vi "SA_Selected_Solution.vi"(7 "Perturbation Method":T1=enum."NonRedundantSwap", 8 "error in (no error)":errorcluster, 9 "Schedule In":u16[](array[numeric]), 10 "GA.lvclass":refnum<class "GA.lvclass">, 11 "OSSP_Problem in":refnum<class "OSSP_Problem.lvclass">) -> (0 "error out":errorcluster, 1 "Schedule Out":u16[](array[numeric]), 2 "OSSP_Problem out":refnum<class "OSSP_Problem.lvclass">, 3 "GA out":refnum<class "GA.lvclass">, 4 "Fitness":i16)   [LabVIEW 2013]
uses:
  Classes/GA.lvclass
  Classes/OSSP_Problem.lvclass
  Classes/SA_Class/Controls/Perturbation Method.ctl
  Classes/SA.lvclass
  SA/Controls/States_SA.ctl
  Classes/OSSP_Problem.lvclass/OSSP_Problem.ctl
  Classes/GA.lvclass/GA.ctl
  Classes/SA_Class/Controls/CoolingScheme.ctl
  Classes/SA.lvclass/SA.ctl
  Classes/SA_Class/Controls/Solution_SA.ctl
  Classes/GanntChart_Class/Operation to Machine Job Tuple.vi
  Classes/GanntChart_Class/Check Other Machines for Schedule Time.vi
  Classes/GanntChart_Class/Schedule Job.vi
  Classes/GanntChart_Class/Find Gaps on Particular Machine.vi
  Classes/GanntChart_Class/Increment Number of Jobs on Machine.vi
  Classes/GanntChart_Class/Find Job On Other Machines.vi
  Classes/GanntChart.lvclass
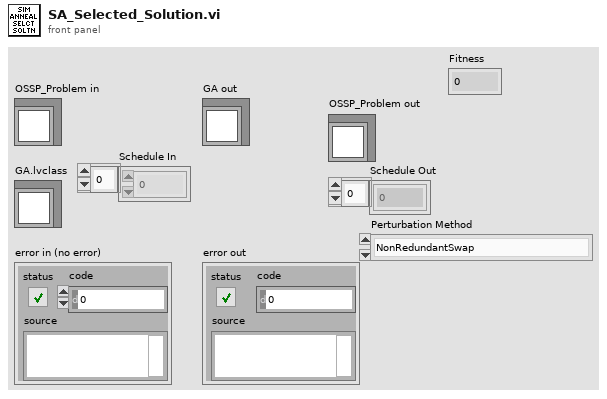
[diagram p1: front panel]
types:
  T1 = typedef "SA.lvclass/Perturbation Method.ctl" = enum16{"Simple Swap", "Insert", "NonRedundantSwap", "Job Order Swap", "Machine Order Swap", "Machine&Job Order Swap", "Critical Path Swap"}
  T2 = typedef "States_SA.ctl" = enum16{"Init", "Read Problem", "Sort Problem", "Generate and Evaluate Current Solution", "Perturb Cur Solution and Eval New Solution", "Make Decision", "Keep Track of Best Solution", "Cool", "Output Final Solution", "Stop"}
  T3 = typedef "Scheduler Type.ctl" = enum16{"Non Delay Scheduler", "GT Active Scheduler", "FIFO Scheduler"}
  T4 = typedef "Objective.ctl" = enum16{"Makespan", "Total Tardiness"}
  T5 = typedef "SA.lvclass/CoolingScheme.ctl" = enum16{"Linear", "Geometric"}
  T6 = typedef "SA.lvclass/Solution_SA.ctl" = cluster{"Schedule":u16[], "Fitness":i16}
  T7 = typedef "GanntChart_Element.ctl" = cluster{"Operation Number":i32, "Job Number":i32, "Start Time":i32, "Procesing Time":u16, "End Time":i32}
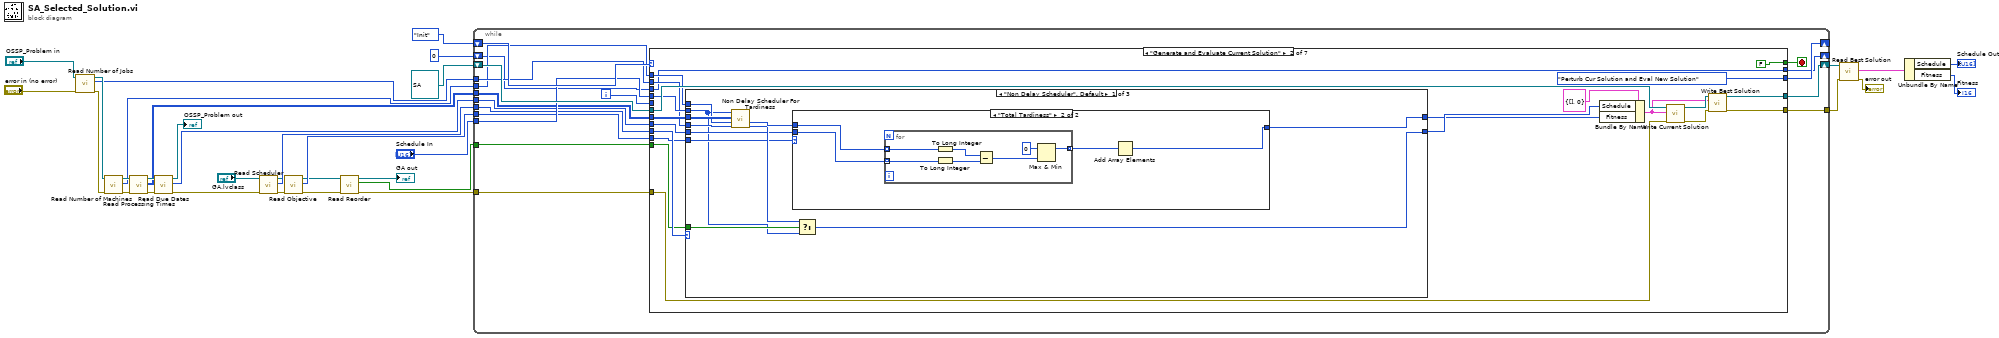
[diagram p0: block diagram]
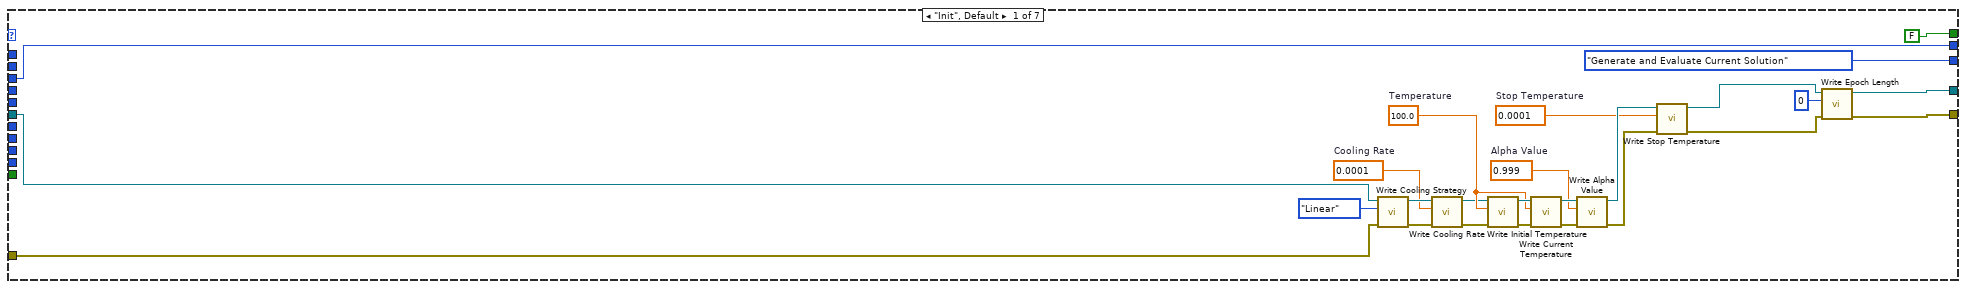
[diagram p2: hidden frame]
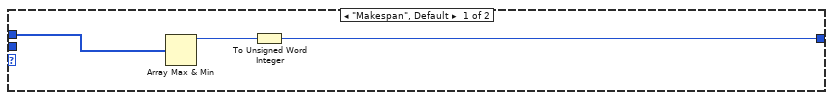
[diagram p3: hidden frame]
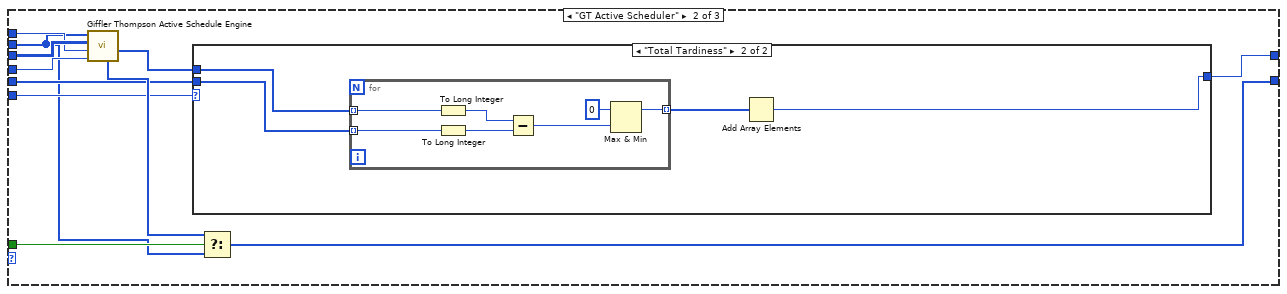
[diagram p4: hidden frame]
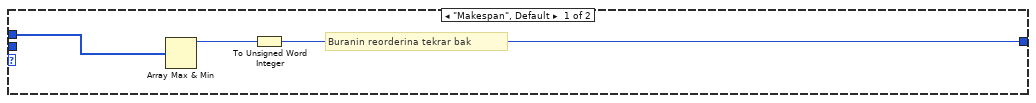
[diagram p5: hidden frame]
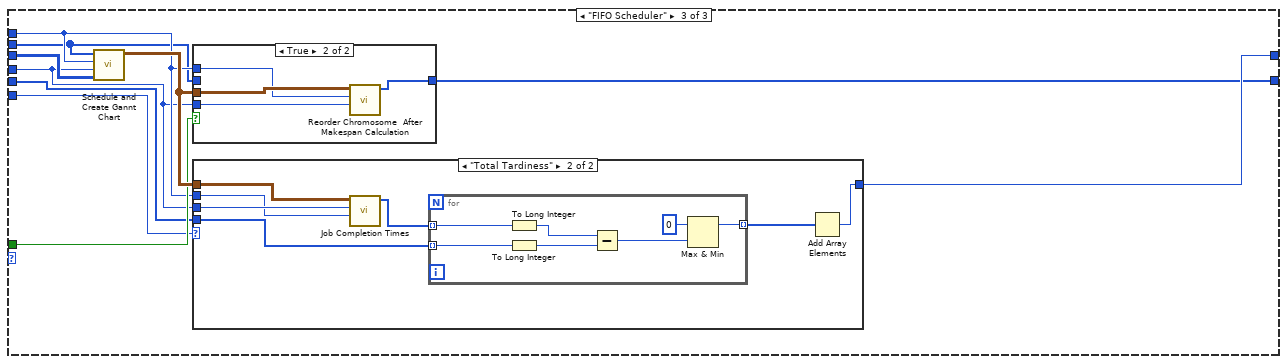
[diagram p6: hidden frame]
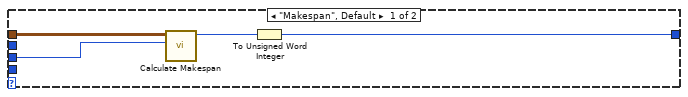
[diagram p8: hidden frame]
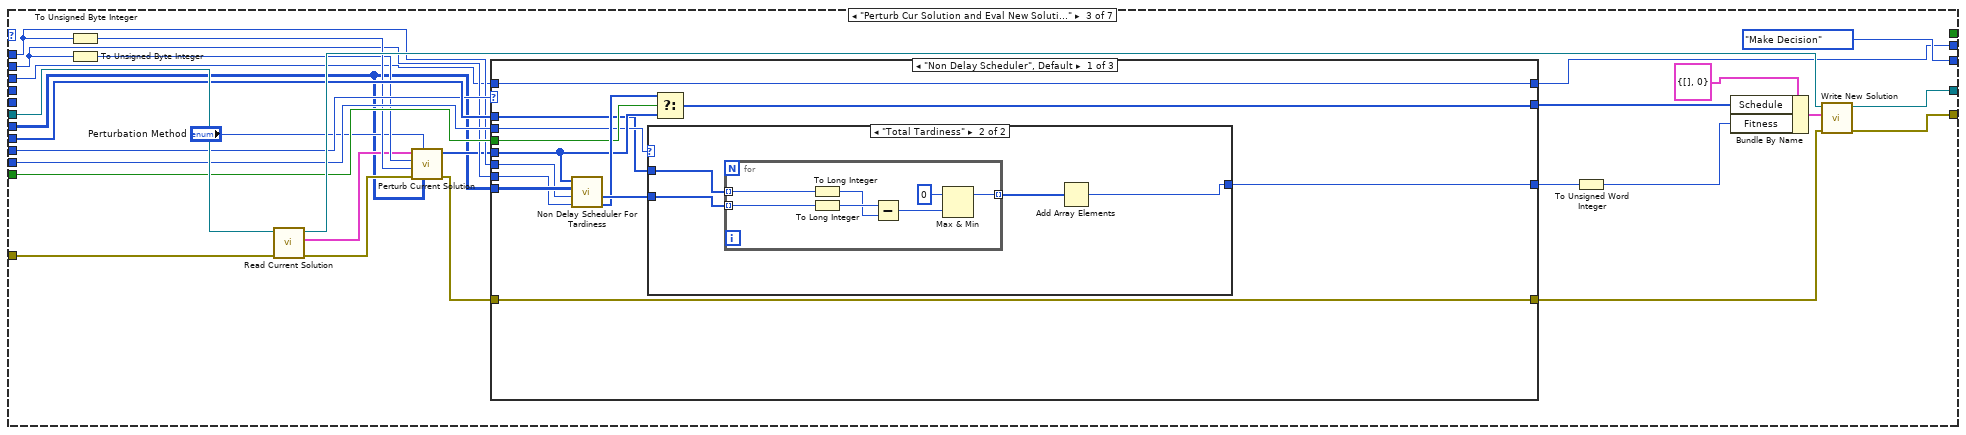
[diagram p9: hidden frame]
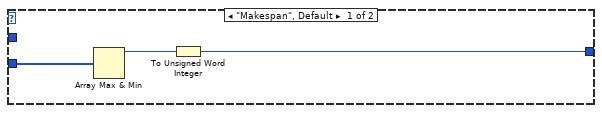
[diagram p10: hidden frame]
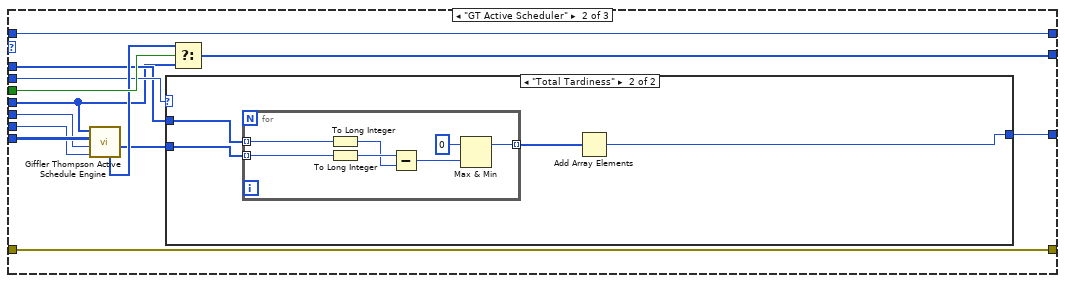
[diagram p11: hidden frame]
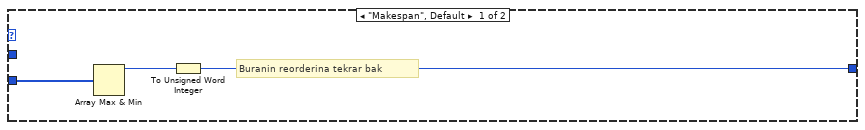
[diagram p12: hidden frame]
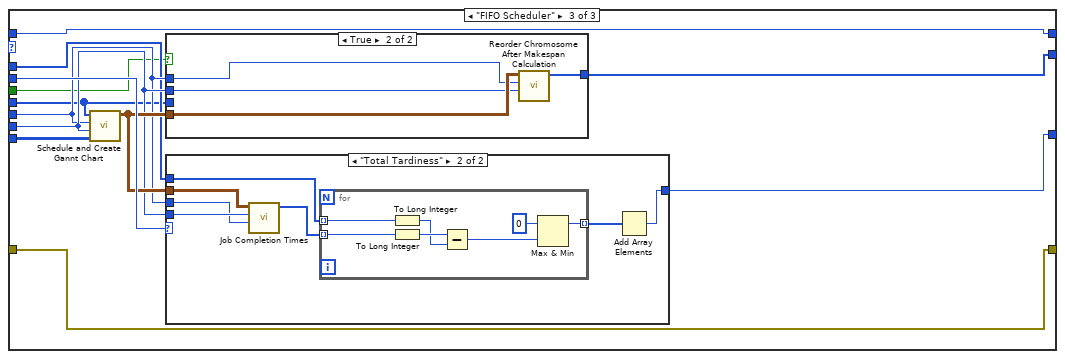
[diagram p13: hidden frame]
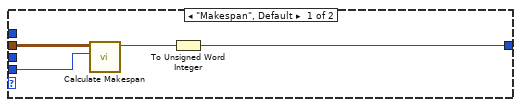
[diagram p15: hidden frame]
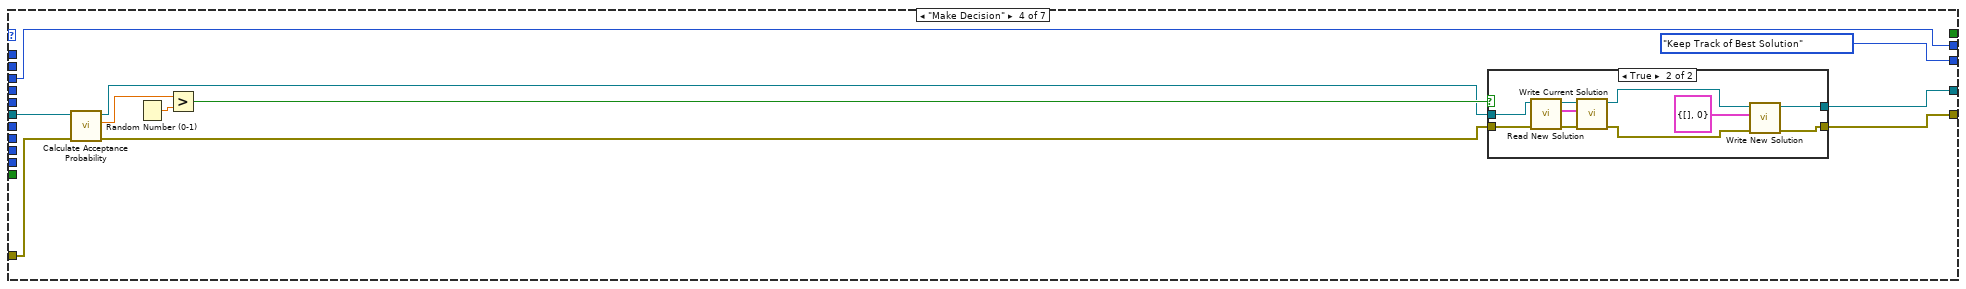
[diagram p16: hidden frame]
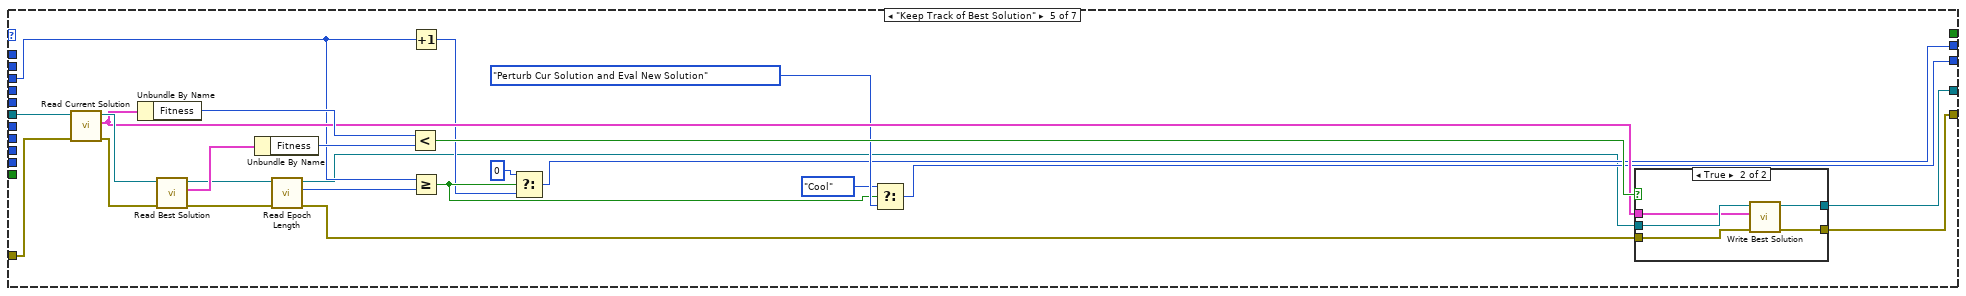
[diagram p18: hidden frame]
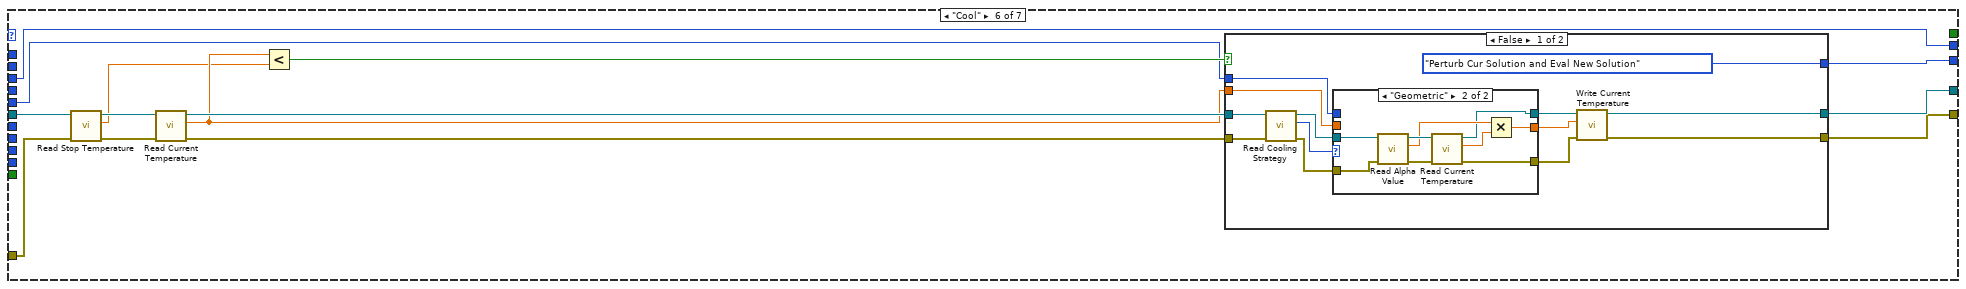
[diagram p20: hidden frame]
diagram:
  n1 = call-dynamic "Read Number of Jobs.vi"("error in (no error)"="error in (no error)", "OSSP_Problem in"="OSSP_Problem in") -> ("error out"=w25:errorcluster, "Number of Jobs"=w29:i32, "OSSP_Problem out"=w31:refnum<class "OSSP_Problem.lvclass">)  [unwired: 7 in]
  n2 = call-dynamic "Read Number of Machines.vi"("error in (no error)"=w25, "OSSP_Problem in"=w31) -> ("error out"=w24:errorcluster, "Number of Machines"=w28:i32, "OSSP_Problem out"=w30:refnum<class "OSSP_Problem.lvclass">)  [unwired: 7 in]
  n3 = call-dynamic "Read Processing Times.vi"("error in (no error)"=w24, "OSSP_Problem in"=w30) -> ("error out"=w23:errorcluster, "Processing Times"=w9:u16[][], "OSSP_Problem out"=w22:refnum<class "OSSP_Problem.lvclass">)  [unwired: 7 in]
  n4 = call "Read Due Dates.vi"("error in (no error)"=w23, "OSSP_Problem in"=w22) -> ("error out"=w20:errorcluster, "Due Dates"=w21:u16[], "OSSP_Problem out"=→"OSSP_Problem out":refnum<class "OSSP_Problem.lvclass">)  [unwired: 7 in]
  n5 = call "Read Scheduler.vi"("error in (no error)"=w20, "GA in"="GA.lvclass") -> ("error out"=w18:errorcluster, "Scheduler"=w19:T3, "GA out"=w17:refnum<class "GA.lvclass">)  [unwired: 7 in]
  n6 = call "Read Objective .vi"("error in (no error)"=w18, "GA in"=w17) -> ("error out"=w15:errorcluster, "Objective"=w16:T4, "GA out"=w12:refnum<class "GA.lvclass">)  [unwired: 7 in]
  n7 = call "Read Reorder.vi"("error in (no error)"=w15, "GA in"=w12) -> ("error out"=w14:errorcluster, "Reorder"=w13:bool, "GA out"=→"GA out":refnum<class "GA.lvclass">)  [unwired: 7 in]
  n8 = while {
    tunnel: "Schedule In" -> [w50]
    shift-right: [w45] -> _
    shift-left: States_SA."Init" ("States") -> [w52]
    tunnel: w29 -> [w49]
    tunnel: w28 -> [w48]
    tunnel: w9 -> [w47]
    shift-right: [w46] -> w27
    shift-left: refnum<class "SA.lvclass"> refnum ("SA.lvclass") -> [w51]
    tunnel: [w43] -> w11
    tunnel: w14 -> [w42]
    tunnel: w21 -> [w41]
    tunnel: w19 -> [w40]
    tunnel: w16 -> [w39]
    tunnel: w13 -> [w38]
    shift-right: [w35] -> _
    shift-left: 0 -> [w36]
    i -> [w37]
    stop <- w44 stop-if-true
    n9 = case shown="\"Generate and Evaluate Current Solution\"" w52 {
      tunnel: w51 -> [w72 w98 w209 w309 w345 w358 w404]
      tunnel: w50 -> [_ w88 _ _ _ _ _]
      tunnel: w49 -> [_ w85 w192 _ _ _ _]
      tunnel: w48 -> [_ w86 w194 _ _ _ _]
      tunnel: w47 -> [_ w87 w184 _ _ _ _]
      tunnel: [w56 w93 w205 w308 w344 w363 w404] -> w46
      tunnel: [States_SA."Generate and Evaluate Current Solution" ("States") States_SA."Perturb Cur Solution and Eval New Solution" ("States") States_SA."Make Decision" ("States") States_SA."Keep Track of Best Solution" w332 w362 States_SA."Stop"] -> w45
      tunnel: [FALSE FALSE _ _ _ _ TRUE] -> w44
      tunnel: [w54 w79 w202 w301 w335 w360 w402] -> w43
      tunnel: w42 -> [w71 w80 w196 w303 w336 w356 w402]
      tunnel: w41 -> [_ w83 w199 _ _ _ _]
      tunnel: w40 -> [_ w91 w198 _ _ _ _]
      tunnel: w39 -> [_ w90 w197 _ _ _ _]
      tunnel: w38 -> [_ w89 w195 _ _ _ _]
      tunnel: w37 -> [_ _ _ _ _ w359 _]
      tunnel: w36 -> [w58 w78 w183 w300 w331 w353 w401]
      tunnel: [w58 w78 w182 w300 w327 w353 w401] -> w35
      frame "Init", Default {
        w64 = 0.0001  # Stop Temperature
        w59 = 0.0001  # Cooling Rate
        w76 = 0.999  # Alpha Value
        w67 = 100.0  # Temperature
        n10 = call "Write Cooling Strategy.vi"("error in (no error)"=w71, "Cooling Strategy"=CoolingScheme."Linear", "SA in"=w72) -> ("error out"=w61:errorcluster, "SA out"=w63:refnum<class "SA.lvclass">)  [unwired: 7 in]
        n11 = call "Write Cooling Rate.vi"("error in (no error)"=w61, "Cooling Rate"=w59, "SA in"=w63) -> ("error out"=w60:errorcluster, "SA out"=w62:refnum<class "SA.lvclass">)  [unwired: 7 in]
        n12 = call "Write Initial Temperature.vi"("error in (no error)"=w60, "Initial Temperature"=w67, "SA in"=w62) -> ("error out"=w68:errorcluster, "SA out"=w69:refnum<class "SA.lvclass">)  [unwired: 7 in]
        n13 = call "Write Current Temperature.vi"("error in (no error)"=w68, "Temperature"=w67, "SA in"=w69) -> ("error out"=w73:errorcluster, "SA out"=w77:refnum<class "SA.lvclass">)  [unwired: 7 in]
        n14 = call "Write Alpha Value.vi"("error in (no error)"=w73, "Alpha Value"=w76, "SA in"=w77) -> ("error out"=w65:errorcluster, "SA out"=w66:refnum<class "SA.lvclass">)  [unwired: 7 in]
        n15 = call "Write Stop Temperature.vi"("error in (no error)"=w65, "Stop Temperature"=w64, "SA in"=w66) -> ("error out"=w55:errorcluster, "SA out"=w57:refnum<class "SA.lvclass">)  [unwired: 7 in]
        n16 = call "Write Epoch Length.vi"("error in (no error)"=w55, "Epoch Length"=u8 0, "SA in"=w57) -> ("error out"=w54:errorcluster, "SA out"=w56:refnum<class "SA.lvclass">)  [unwired: 7 in]
      }
      frame "Generate and Evaluate Current Solution" {
        n17 = case shown="\"Non Delay Scheduler\", Default" w91 {
          tunnel: [w105 w130 w158] -> w82
          tunnel: [w106 w131 w156] -> w84
          tunnel: w88 -> [w99 w124 w149]
          tunnel: w89 -> [w107 w134 w155]
          tunnel: w90 -> [w104 w127 w152]
          tunnel: w87 -> [w103 w129 w154]
          tunnel: w86 -> [w102 w126 w151]
          tunnel: w85 -> [w101 w125 w150]
          tunnel: w83 -> [w100 w128 w153]
          frame "Non Delay Scheduler", Default {
            n18 = call "Non Delay Scheduler For Tardiness.vi"("Number of  Jobs"=w101, "Number of Machines"=w102, "Processing Times"=w103, "Schedule"=w99) -> ("Scheduled Jobs Order"=w108:u16[], "Job Completion Times"=w109:u16[])  [unwired: 3 in, 3 out]
            n19 = case shown="\"Total Tardiness\"" w104 {
              tunnel: w109 -> [w112 w116]
              tunnel: [w110 w113] -> w105
              tunnel: w100 -> [_ w115]
              frame "Makespan", Default {
                n20 = Array Max & Min(array=w112) -> (max value=w111:u16)  [unwired: 3 out]
                n21 = To Unsigned Word Integer(number=w111) -> (unsigned 16bit integer=w110:u16)
              }
              frame "Total Tardiness" {
                n22 = for {
                  tunnel: w116 -> [w123] mode=indexing
                  tunnel: w115 -> [w122] mode=indexing
                  tunnel: [w117] -> w114 mode=indexing
                  n23 = To Long Integer(number=w123) -> (32bit integer=w121:i32)
                  n24 = To Long Integer(number=w122) -> (32bit integer=w120:i32)
                  n25 = Subtract(x=w121, y=w120) -> (x-y=w119:i32)
                  n26 = Max & Min(x=0, y=w119) -> (max(x,y)=w117:i32)  [unwired: 1 out]
                }
                n27 = Add Array Elements(numeric array=w114) -> (sum=w113:i32)
              }
            }
            n28 = Select(t=w108, s=w107, f=w99) -> (s? t:f=w106:u16[])
          }
          frame "GT Active Scheduler" {
            n29 = call "Giffler Thompson Active Schedule Engine.vi"("Number of  Jobs"=w125, "Number of Machines"=w126, "Processing Times"=w129, "Schedule In"=w124) -> ("Job Completion Times"=w132:u16[], "Schedule Order"=w133:u16[])  [unwired: 3 in, 3 out]
            n30 = case shown="\"Total Tardiness\"" w127 {
              tunnel: w132 -> [w137 w140]
              tunnel: [w135 w138] -> w130
              tunnel: w128 -> [_ w139]
              frame "Makespan", Default {
                # "Buranin reorderina tekrar bak"
                n31 = Array Max & Min(array=w137) -> (max value=w136:u16)  [unwired: 3 out]
                n32 = To Unsigned Word Integer(number=w136) -> (unsigned 16bit integer=w135:u16)
              }
              frame "Total Tardiness" {
                n33 = for {
                  tunnel: [w144] -> w141 mode=indexing
                  tunnel: w140 -> [w143] mode=indexing
                  tunnel: w139 -> [w142] mode=indexing
                  n34 = To Long Integer(number=w143) -> (32bit integer=w148:i32)
                  n35 = To Long Integer(number=w142) -> (32bit integer=w147:i32)
                  n36 = Subtract(x=w148, y=w147) -> (x-y=w146:i32)
                  n37 = Max & Min(x=0, y=w146) -> (max(x,y)=w144:i32)  [unwired: 1 out]
                }
                n38 = Add Array Elements(numeric array=w141) -> (sum=w138:i32)
              }
            }
            n39 = Select(t=w133, s=w134, f=w124) -> (s? t:f=w131:u16[])
          }
          frame "FIFO Scheduler" {
            n40 = call "Schedule and Create Gannt Chart.vi"("Processing Times (Rows Mach.Cols Jobs)"=w154, "Number of Jobs"=w150, "Number of Machines"=w151, "Schedule"=w149) -> ("Gannt Chart Out"=w157:T7[][])  [unwired: 6 in, 1 out]
            n41 = case shown="True" w155 {
              tunnel: w157 -> [_ w163]
              tunnel: [w159 w162] -> w156
              tunnel: w151 -> [_ w161]
              tunnel: w150 -> [_ w160]
              tunnel: w149 -> [w159 _]
              frame False {
              }
              frame True {
                n42 = call "Reorder Chromosome  After Makespan Calculation.vi"("Number Of  Jobs"=w160, "Number Of Machines"=w161, "Gannt Chart In"=w163) -> ("Reordered Chromosome"=w162:u16[])  [unwired: 8 in]
              }
            }
            n43 = case shown="\"Total Tardiness\"" w152 {
              tunnel: w157 -> [w167 w174]
              tunnel: [w165 w168] -> w158
              tunnel: w153 -> [_ w169]
              tunnel: w150 -> [w164 w173]
              tunnel: w151 -> [_ w172]
              frame "Makespan", Default {
                n44 = call "Calculate Makespan.vi"("Number of Jobs"=w164, "Gannt Chart In"=w167) -> ("Makespan"=w166:i32)  [unwired: 9 in]
                n45 = To Unsigned Word Integer(number=w166) -> (unsigned 16bit integer=w165:u16)
              }
              frame "Total Tardiness" {
                n46 = call "Job Completion Times.vi"("Number Of Machines"=w172, "Number Of Jobs"=w173, "Gannt Chart In"=w174) -> ("Job Completion Times"=w170:u16[])  [unwired: 8 in]
                n47 = for {
                  tunnel: [w177] -> w171 mode=indexing
                  tunnel: w170 -> [w176] mode=indexing
                  tunnel: w169 -> [w175] mode=indexing
                  n48 = To Long Integer(number=w176) -> (32bit integer=w181:i32)
                  n49 = To Long Integer(number=w175) -> (32bit integer=w180:i32)
                  n50 = Subtract(x=w181, y=w180) -> (x-y=w179:i32)
                  n51 = Max & Min(x=0, y=w179) -> (max(x,y)=w177:i32)  [unwired: 1 out]
                }
                n52 = Add Array Elements(numeric array=w171) -> (sum=w168:i32)
              }
            }
          }
        }
        n53 = Bundle By Name(cluster=T6 {"Schedule"=[], "Fitness"=0} ("Solution"), "Schedule"=w84, "Fitness"=w82) -> (w92:T6)
        n54 = call "Write Current Solution.vi"("error in (no error)"=w80, "Solution"=w92, "SA in"=w98) -> ("error out"=w81:errorcluster, "SA out"=w94:refnum<class "SA.lvclass">)  [unwired: 7 in]
        n55 = call "Write Best Solution.vi"("error in (no error)"=w81, "Solution"=w92, "SA in"=w94) -> ("error out"=w79:errorcluster, "SA out"=w93:refnum<class "SA.lvclass">)  [unwired: 7 in]
      }
      frame "Perturb Cur Solution and Eval New Solution" {
        n56 = To Unsigned Byte Integer(number=w194) -> (unsigned 8bit integer=w193:u8)
        n57 = To Unsigned Byte Integer(number=w192) -> (unsigned 8bit integer=w191:u8)
        n58 = call "Read Current Solution.vi"("error in (no error)"=w196, "SA in"=w209) -> ("error out"=w189:errorcluster, "Solution"=w185:T6, "SA out"=w208:refnum<class "SA.lvclass">)  [unwired: 7 in]
        n59 = call "Perturb Current Solution.vi"("Processing Times (Rows Machine, Columns Jobs)"=w184, "Perturbation Method"="Perturbation Method", "error in (no error)"=w189, "Number of Machines"=w193, "Number of Jobs"=w191, "Solution"=w185) -> ("error out"=w188:errorcluster, "Perturbed Schedule"=w186:u16[])  [unwired: 4 in]
        n60 = case shown="\"Non Delay Scheduler\", Default" w198 {
          tunnel: w186 -> [w216 w241 w266]
          tunnel: w194 -> [w218 w243 w269]
          tunnel: w192 -> [w219 w245 w271]
          tunnel: w184 -> [w220 w249 w275]
          tunnel: [w212 w239 w274] -> w201
          tunnel: w197 -> [w214 w244 w273]
          tunnel: [w215 w240 w270] -> w200
          tunnel: w199 -> [w213 w242 w268]
          tunnel: w195 -> [w217 w248 w267]
          tunnel: [w211 w238 w265] -> w187
          tunnel: w188 -> [w211 w238 w265]
          tunnel: w183 -> [w210 w237 w264]
          tunnel: [w210 w237 w264] -> w182
          frame "Non Delay Scheduler", Default {
            n61 = call "Non Delay Scheduler For Tardiness.vi"("Number of  Jobs"=w219, "Number of Machines"=w218, "Processing Times"=w220, "Schedule"=w216) -> ("Scheduled Jobs Order"=w221:u16[], "Job Completion Times"=w222:u16[])  [unwired: 3 in, 3 out]
            n62 = case shown="\"Total Tardiness\"" w214 {
              tunnel: w222 -> [w225 w228]
              tunnel: [w223 w226] -> w212
              tunnel: w213 -> [_ w227]
              frame "Makespan", Default {
                n63 = Array Max & Min(array=w225) -> (max value=w224:u16)  [unwired: 3 out]
                n64 = To Unsigned Word Integer(number=w224) -> (unsigned 16bit integer=w223:u16)
              }
              frame "Total Tardiness" {
                n65 = for {
                  tunnel: w228 -> [w236] mode=indexing
                  tunnel: w227 -> [w235] mode=indexing
                  tunnel: [w230] -> w229 mode=indexing
                  n66 = To Long Integer(number=w235) -> (32bit integer=w233:i32)
                  n67 = To Long Integer(number=w236) -> (32bit integer=w234:i32)
                  n68 = Subtract(x=w234, y=w233) -> (x-y=w232:i32)
                  n69 = Max & Min(x=0, y=w232) -> (max(x,y)=w230:i32)  [unwired: 1 out]
                }
                n70 = Add Array Elements(numeric array=w229) -> (sum=w226:i32)
              }
            }
            n71 = Select(t=w221, s=w217, f=w216) -> (s? t:f=w215:u16[])
          }
          frame "GT Active Scheduler" {
            n72 = call "Giffler Thompson Active Schedule Engine.vi"("Number of  Jobs"=w245, "Number of Machines"=w243, "Processing Times"=w249, "Schedule In"=w241) -> ("Job Completion Times"=w246:u16[], "Schedule Order"=w247:u16[])  [unwired: 3 in, 3 out]
            n73 = case shown="\"Total Tardiness\"" w244 {
              tunnel: w246 -> [w252 w255]
              tunnel: [w250 w253] -> w239
              tunnel: w242 -> [_ w254]
              frame "Makespan", Default {
                # "Buranin reorderina tekrar bak"
                n74 = Array Max & Min(array=w252) -> (max value=w251:u16)  [unwired: 3 out]
                n75 = To Unsigned Word Integer(number=w251) -> (unsigned 16bit integer=w250:u16)
              }
              frame "Total Tardiness" {
                n76 = for {
                  tunnel: [w259] -> w256 mode=indexing
                  tunnel: w255 -> [w258] mode=indexing
                  tunnel: w254 -> [w257] mode=indexing
                  n77 = To Long Integer(number=w257) -> (32bit integer=w262:i32)
                  n78 = To Long Integer(number=w258) -> (32bit integer=w263:i32)
                  n79 = Subtract(x=w263, y=w262) -> (x-y=w261:i32)
                  n80 = Max & Min(x=0, y=w261) -> (max(x,y)=w259:i32)  [unwired: 1 out]
                }
                n81 = Add Array Elements(numeric array=w256) -> (sum=w253:i32)
              }
            }
            n82 = Select(t=w247, s=w248, f=w241) -> (s? t:f=w240:u16[])
          }
          frame "FIFO Scheduler" {
            n83 = call "Schedule and Create Gannt Chart.vi"("Processing Times (Rows Mach.Cols Jobs)"=w275, "Number of Jobs"=w271, "Number of Machines"=w269, "Schedule"=w266) -> ("Gannt Chart Out"=w272:T7[][])  [unwired: 6 in, 1 out]
            n84 = case shown="True" w267 {
              tunnel: w272 -> [_ w280]
              tunnel: w269 -> [_ w279]
              tunnel: w271 -> [_ w278]
              tunnel: [w276 w277] -> w270
              tunnel: w266 -> [w276 _]
              frame False {
              }
              frame True {
                n85 = call "Reorder Chromosome  After Makespan Calculation.vi"("Number Of  Jobs"=w278, "Number Of Machines"=w279, "Gannt Chart In"=w280) -> ("Reordered Chromosome"=w277:u16[])  [unwired: 8 in]
              }
            }
            n86 = case shown="\"Total Tardiness\"" w273 {
              tunnel: w272 -> [w284 w291]
              tunnel: [w281 w285] -> w274
              tunnel: w271 -> [w283 w290]
              tunnel: w269 -> [_ w289]
              tunnel: w268 -> [_ w286]
              frame "Makespan", Default {
                n87 = call "Calculate Makespan.vi"("Number of Jobs"=w283, "Gannt Chart In"=w284) -> ("Makespan"=w282:i32)  [unwired: 9 in]
                n88 = To Unsigned Word Integer(number=w282) -> (unsigned 16bit integer=w281:u16)
              }
              frame "Total Tardiness" {
                n89 = call "Job Completion Times.vi"("Number Of Machines"=w289, "Number Of Jobs"=w290, "Gannt Chart In"=w291) -> ("Job Completion Times"=w287:u16[])  [unwired: 8 in]
                n90 = for {
                  tunnel: [w294] -> w288 mode=indexing
                  tunnel: w287 -> [w293] mode=indexing
                  tunnel: w286 -> [w292] mode=indexing
                  n91 = To Long Integer(number=w292) -> (32bit integer=w297:i32)
                  n92 = To Long Integer(number=w293) -> (32bit integer=w298:i32)
                  n93 = Subtract(x=w298, y=w297) -> (x-y=w296:i32)
                  n94 = Max & Min(x=0, y=w296) -> (max(x,y)=w294:i32)  [unwired: 1 out]
                }
                n95 = Add Array Elements(numeric array=w288) -> (sum=w285:i32)
              }
            }
          }
        }
        n96 = To Unsigned Word Integer(number=w201) -> (unsigned 16bit integer=w203:u16)
        n97 = Bundle By Name(cluster=T6 {"Schedule"=[], "Fitness"=0} ("Solution"), "Schedule"=w200, "Fitness"=w203) -> (w206:T6)
        n98 = call "Write New Solution.vi"("error in (no error)"=w187, "Solution"=w206, "SA in"=w208) -> ("error out"=w202:errorcluster, "SA out"=w205:refnum<class "SA.lvclass">)  [unwired: 7 in]
      }
      frame "Make Decision" {
        n99 = call "Calculate Acceptance Probability.vi"("error in (no error)"=w303, "SA in"=w309) -> ("error out"=w302:errorcluster, "Acceptance Probability"=w307:dbl, "SA out"=w304:refnum<class "SA.lvclass">)  [unwired: 7 in]
        n100 = Random Number (0-1)() -> (number: 0 to 1=w306:dbl)
        n101 = Greater?(x=w307, y=w306) -> (0:w305:bool)
        n102 = case shown="True" w305 {
          tunnel: w304 -> [w311 w321]
          tunnel: [w311 w315] -> w308
          tunnel: w302 -> [w310 w314]
          tunnel: [w310 w313] -> w301
          frame False {
          }
          frame True {
            n103 = call "Read New Solution.vi"("error in (no error)"=w314, "SA in"=w321) -> ("error out"=w320:errorcluster, "Solution"=w318:T6, "SA out"=w319:refnum<class "SA.lvclass">)  [unwired: 7 in]
            n104 = call "Write Current Solution.vi"("error in (no error)"=w320, "Solution"=w318, "SA in"=w319) -> ("error out"=w316:errorcluster, "SA out"=w317:refnum<class "SA.lvclass">)  [unwired: 7 in]
            n105 = call "Write New Solution.vi"("error in (no error)"=w316, "Solution"=T6 {"Schedule"=[], "Fitness"=0}, "SA in"=w317) -> ("error out"=w313:errorcluster, "SA out"=w315:refnum<class "SA.lvclass">)  [unwired: 7 in]
          }
        }
      }
      frame "Keep Track of Best Solution" {
        n106 = call "Read Current Solution.vi"("error in (no error)"=w336, "SA in"=w345) -> ("error out"=w337:errorcluster, "Solution"=w338:T6, "SA out"=w343:refnum<class "SA.lvclass">)  [unwired: 7 in]
        n107 = Unbundle By Name(w338) -> ("Fitness"=w342:i16)
        n108 = call "Read Best Solution.vi"("error in (no error)"=w337, "SA in"=w343) -> ("error out"=w323:errorcluster, "Solution"=w341:T6, "SA out"=w326:refnum<class "SA.lvclass">)  [unwired: 7 in]
        n109 = Unbundle By Name(w341) -> ("Fitness"=w340:i16)
        n110 = call "Read Epoch Length.vi"("error in (no error)"=w323, "SA in"=w326) -> ("error out"=w322:errorcluster, "Epoch Length"=w324:u8, "SA out"=w325:refnum<class "SA.lvclass">)  [unwired: 7 in]
        n111 = Less?(x=w342, y=w340) -> (x < y?=w339:bool)
        n112 = Increment(x=w331) -> (x+1=w329:i32)
        n113 = Greater Or Equal?(x=w331, y=w324) -> (x >= y?=w330:bool)
        n114 = Select(t=0, s=w330, f=w329) -> (s? t:f=w327:i32)
        n115 = Select(t=States_SA."Cool", s=w330, f=States_SA."Perturb Cur Solution and Eval New Solution") -> (s? t:f=w332:T2)
        n116 = case shown="True" w339 {
          tunnel: w325 -> [w347 w352]
          tunnel: [w347 w351] -> w344
          tunnel: w338 -> [_ w350]
          tunnel: w322 -> [w346 w349]
          tunnel: [w346 w348] -> w335
          frame False {
          }
          frame True {
            n117 = call "Write Best Solution.vi"("error in (no error)"=w349, "Solution"=w350, "SA in"=w352) -> ("error out"=w348:errorcluster, "SA out"=w351:refnum<class "SA.lvclass">)  [unwired: 7 in]
          }
        }
      }
      frame "Cool" {
        n118 = call "Read Stop Temperature.vi"("error in (no error)"=w356, "SA in"=w358) -> ("error out"=w355:errorcluster, "Stop Temperature"=w354:dbl, "SA out"=w357:refnum<class "SA.lvclass">)  [unwired: 7 in]
        n119 = call "Read Current Temperature.vi"("error in (no error)"=w355, "SA in"=w357) -> ("error out"=w361:errorcluster, "Temperature"=w364:dbl, "SA out"=w365:refnum<class "SA.lvclass">)  [unwired: 7 in]
        n120 = Less?(x=w364, y=w354) -> (x < y?=w366:bool)
        n121 = case shown="False" w366 {
          tunnel: [States_SA."Perturb Cur Solution and Eval New Solution" ("f") States_SA."Stop"] -> w362
          tunnel: w365 -> [w372 w399]
          tunnel: [w378 w399] -> w363
          tunnel: w364 -> [w374 _]
          tunnel: w361 -> [w370 w398]
          tunnel: [w373 w398] -> w360
          tunnel: w359 -> [w367 _]
          frame False {
            n122 = call "Read Cooling Strategy.vi"("error in (no error)"=w370, "SA in"=w372) -> ("error out"=w369:errorcluster, "Cooling Strategy"=w368:T5, "SA out"=w371:refnum<class "SA.lvclass">)  [unwired: 7 in]
            n123 = case shown="\"Geometric\"" w368 {
              tunnel: w371 -> [w388 w397]
              tunnel: [w387 w389] -> w377
              tunnel: [w386 w392] -> w376
              tunnel: [w382 w395] -> w375
              tunnel: w374 -> [w381 _]
              tunnel: w369 -> [w380 w396]
              tunnel: w367 -> [_ _]
              frame "Linear", Default {
                n124 = call "Read Cooling Rate.vi"("error in (no error)"=w380, "SA in"=w388) -> ("error out"=w386:errorcluster, "Cooling Rate"=w384:dbl, "SA out"=w387:refnum<class "SA.lvclass">)  [unwired: 7 in]
                n125 = Subtract(x=1.0, y=w384) -> (x-y=w383:dbl)
                n126 = Multiply(x=w383, y=w381) -> (x*y=w382:dbl)
              }
              frame "Geometric" {
                n127 = call "Read Alpha Value.vi"("error in (no error)"=w396, "SA in"=w397) -> ("error out"=w393:errorcluster, "Alpha Value"=w391:dbl, "SA out"=w394:refnum<class "SA.lvclass">)  [unwired: 7 in]
                n128 = call "Read Current Temperature.vi"("error in (no error)"=w393, "SA in"=w394) -> ("error out"=w392:errorcluster, "Temperature"=w390:dbl, "SA out"=w389:refnum<class "SA.lvclass">)  [unwired: 7 in]
                n129 = Multiply(x=w391, y=w390) -> (x*y=w395:dbl)
              }
            }
            n130 = call "Write Current Temperature.vi"("error in (no error)"=w376, "Temperature"=w375, "SA in"=w377) -> ("error out"=w373:errorcluster, "SA out"=w378:refnum<class "SA.lvclass">)  [unwired: 7 in]
          }
          frame True {
          }
        }
      }
      frame "Stop" {
      }
    }
  }
  n131 = call "Read Best Solution.vi"("error in (no error)"=w11, "SA in"=w27) -> ("error out"=→"error out":errorcluster, "Solution"=w26:T6)  [unwired: 7 in, 1 out]
  n132 = Unbundle By Name(w26) -> ("Schedule"=→"Schedule Out":u16[], "Fitness"=→"Fitness":i16)
